vi "Cycle 0 Coast to Zero.vi"(0 "GEA2 Reference In":refnum<k24>, 5 "GEA Inputs":T1 {"Destination" format="%.0x"; "Source" format="%.0x"}, 7 "Standalone?":bool, 11 "Error In":errorcluster) -> (4 "GEA2 Reference Out":refnum<k24>, 6 "Pass/Fail?":bool, 8 "Report Text":string, 15 "Error Out":errorcluster)   [LabVIEW 2016, in "2015 VA Washer.lvlib"]
uses:
  Projects/2015 VA Washer.lvlib
  C:/Automation/DLLs/PC Dot Net/GeaCommunication.dll
  Common/LabVIEW GEA2 Toolkit/LabVIEW_GEA2_Toolkit.lvlibp/type defs/Source_Destination.ctl
  Valew Common/type defs/Drive Cycle Engine Request State.ctl
  Common/LabVIEW GEA2 Toolkit/LabVIEW_GEA2_Toolkit.lvlibp/type defs/ERD Read Data In.ctl
  Common/LabVIEW GEA2 Toolkit/LabVIEW_GEA2_Toolkit.lvlibp/type defs/Data Type.ctl
  Common/LabVIEW GEA2 Toolkit/LabVIEW_GEA2_Toolkit.lvlibp
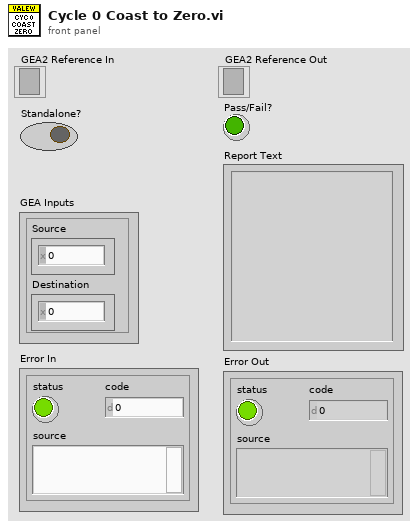
[diagram p1: front panel]
types:
  T1 = typedef "LabVIEW_GEA2_Toolkit.lvlibp/Source_Destination.ctl" = cluster{"Source":u8, "Destination":u8}
  T2 = typedef "2015 VA Washer.lvlib/Drive Cycle Engine Request State.ctl" = enum16{"Start", "Stop", "Pause", "Resume", "Select"}
  T3 = typedef "LabVIEW_GEA2_Toolkit.lvlibp/ERD Read Data In.ctl" = cluster{"ERD Number":u16, "Data Type":T4}
  T4 = typedef "LabVIEW_GEA2_Toolkit.lvlibp/Data Type.ctl" = enum16{"string", "boolean", "uint8_t", "uint16_t", "uint32_t", "uint64_t", "int8_t", "int16_t", "int32_t", "int64_t"}
  T5 = typedef "LabVIEW_GEA2_Toolkit.lvlibp/ERD Read Data Out.ctl" = cluster{"ERD Number":u16, "Data":string}
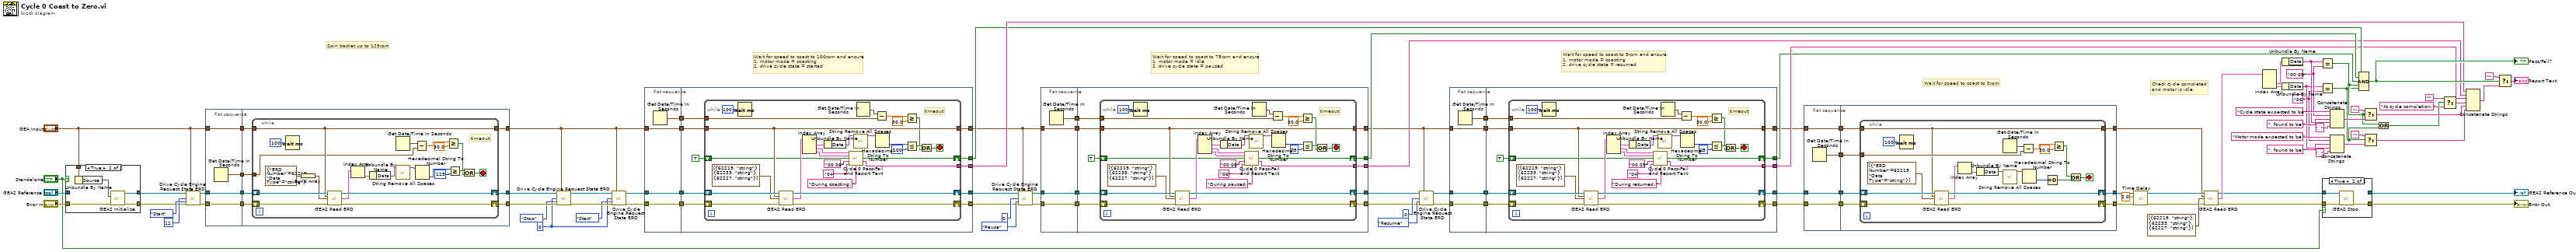
[diagram p0: block diagram]
diagram:
  w80 = "00 0B" ("y")
  w70 = "06" ("y")
  w93 = u8 0 ("Cycle ID")
  # "Check cycle completed\nand motor is idle"
  # "Wait for speed to coast to 0rpm"
  # "Wait for speed to coast to 5rpm and ensure\n1. motor mode = coasting\n2. drive cycle state = resumed"
  # "Wait for speed to coast to 75rpm and ensure\n1. motor mode = idle\n2. drive cycle state = paused"
  # "Wait for speed to coast to 100rpm and ensure\n1. motor mode = coasting\n2. drive cycle state = started"
  # "Spin basket up to 125rpm"
  n1 = case shown="True" "Standalone?" {
    tunnel: "GEA2 Reference In" -> [w104 _]
    tunnel: [w104 w109] -> w19
    tunnel: "Error In" -> [w103 w108]
    tunnel: [w103 w107] -> w17
    tunnel: "GEA Inputs" -> [_ w106]
    frame False {
    }
    frame True {
      n2 = Unbundle By Name(w106) -> ("Source"=w105:u8)
      n3 = call "GEA2 Initialize.vi"("Source Address"=w105, "error in"=w108) -> ("GEA2 Reference Out"=w109:refnum<k24>, "error out"=w107:errorcluster)  [unwired: 11 in, 1 out]
    }
  }
  n4 = call "Drive Cycle Engine Request State ERD.vi"("GEA2 Reference In"=w19, "GEA Inputs"="GEA Inputs", "Cycle ID"=u8 12, "Drive Cycle Engine Request State"=Drive_Cycle_Engine_Request_State."Start", "Error In"=w17) -> ("GEA2 Reference Out"=w99:refnum<k24>, "Error Out"=w100:errorcluster)  [unwired: 9 in]
  n5 = flat-sequence {
    tunnel: "GEA Inputs" -> [w111]
    tunnel: w99 -> [w112]
    tunnel: w100 -> [w113]
    tunnel: [w113] -> w91
    tunnel: [w112] -> w90
    tunnel: [w111] -> w89
    tunnel: [w110] -> w88
    tunnel: [w118] -> w98
    tunnel: [w117] -> w97
    tunnel: [w115] -> w49
    tunnel: w91 -> [w120]
    tunnel: w90 -> [w119]
    tunnel: w89 -> [w116]
    tunnel: w88 -> [w114]
    frame #0 {
      n6 = Get Date/Time In Seconds() -> (seconds since 1Jan1904=w110:timestamp)
    }
    frame #1 {
      n7 = while {
        shift-right: [w140] -> w117
        shift-left: w120 -> [w141]
        shift-right: [w138] -> w118
        shift-left: w119 -> [w139]
        tunnel: w116 -> [w131]
        tunnel: [w131] -> w115
        tunnel: w114 -> [w129]
        stop <- w126 stop-if-true
        # "timeout"
        n8 = Wait (ms)(milliseconds to wait=u32 100) -> ()  [unwired: 1 out]
        n9 = Build Array(T3 {"ERD Number"=62219, "Data Type"=enum."string"} ("ERD Read Data In")) -> (w137:T3[])
        n10 = call "GEA2 Read ERD.vi"("GEA2 Reference In"=w139, "GEA Inputs"=w131, "Read ERD List"=w137, "Error In"=w141) -> ("GEA2 Reference Out"=w138:refnum<k24>, "ERD Data Out"=w135:T5[], "Error Out"=w140:errorcluster)  [unwired: 8 in, 1 out]
        n11 = Index Array(array=w135) -> (element=w134:T5)  [unwired: 1 in]
        n12 = Unbundle By Name(w134) -> ("Data"=w121:string)
        n13 = Get Date/Time In Seconds() -> (seconds since 1Jan1904=w130:timestamp)
        n14 = call "String Remove All Spaces.vi"("Input String"=w121) -> ("Spaces Removed"=w122:string)  [unwired: 13 in, 1 out]
        n15 = Subtract(x=w130, y=w129) -> (x-y=w128:dbl)
        n16 = Hexadecimal String To Number(string=w122) -> (number=w133:u32)  [unwired: 2 in, 1 out]
        n17 = Greater Or Equal?(x=w128, y=30.0) -> (x >= y?=w124:bool)
        n18 = Greater Or Equal?(x=w133, y=u32 125) -> (x >= y?=w125:bool)
        n19 = Or(x=w125, y=w124) -> (x .or. y?=w126:bool)
      }
    }
  }
  n20 = call "Drive Cycle Engine Request State ERD.vi"("GEA2 Reference In"=w98, "GEA Inputs"=w49, "Cycle ID"=w93, "Drive Cycle Engine Request State"=Drive_Cycle_Engine_Request_State."Stop", "Error In"=w97) -> ("GEA2 Reference Out"=w95:refnum<k24>, "Error Out"=w94:errorcluster)  [unwired: 9 in]
  n21 = call "Drive Cycle Engine Request State ERD.vi"("GEA2 Reference In"=w95, "GEA Inputs"=w49, "Cycle ID"=w93, "Drive Cycle Engine Request State"=Drive_Cycle_Engine_Request_State."Start", "Error In"=w94) -> ("GEA2 Reference Out"=w50:refnum<k24>, "Error Out"=w51:errorcluster)  [unwired: 9 in]
  n22 = flat-sequence {
    tunnel: w51 -> [w143]
    tunnel: w49 -> [w144]
    tunnel: w50 -> [w145]
    tunnel: [w145] -> w55
    tunnel: [w144] -> w54
    tunnel: [w143] -> w53
    tunnel: [w142] -> w52
    tunnel: w55 -> [w155]
    tunnel: w54 -> [w154]
    tunnel: w53 -> [w153]
    tunnel: w52 -> [w152]
    tunnel: [w150] -> w47
    tunnel: [w149] -> w48
    tunnel: [w148] -> w38
    tunnel: [w147] -> w45
    tunnel: [w146] -> w46
    frame #0 {
      n23 = Get Date/Time In Seconds() -> (seconds since 1Jan1904=w142:timestamp)
    }
    frame #1 {
      n24 = while {
        shift-right: [w182] -> w150
        shift-left: w153 -> [w183]
        shift-right: [w180] -> w149
        shift-left: w155 -> [w181]
        tunnel: w154 -> [w177]
        tunnel: [w177] -> w148
        tunnel: w152 -> [w174]
        shift-right: [w160] -> w147
        shift-left: TRUE -> [w161]
        tunnel: [w159] -> w146
        stop <- w171 stop-if-true
        # "timeout"
        n25 = Wait (ms)(milliseconds to wait=u32 100) -> ()  [unwired: 1 out]
        n26 = call "GEA2 Read ERD.vi"("GEA2 Reference In"=w181, "GEA Inputs"=w177, "Read ERD List"=T3[] [{"ERD Number"=62219, "Data Type"=enum."string"}, {"ERD Number"=62233, "Data Type"=enum."string"}, {"ERD Number"=62227, "Data Type"=enum."string"}], "Error In"=w183) -> ("GEA2 Reference Out"=w180:refnum<k24>, "ERD Data Out"=w179:T5[], "Error Out"=w182:errorcluster)  [unwired: 8 in, 1 out]
        n27 = Index Array(array=w179) -> (element #1=w178:T5, element #2=w163:T5, element #3=w162:T5)  [unwired: 3 in]
        n28 = Unbundle By Name(w178) -> ("Data"=w166:string)
        n29 = call "Cycle 0 Pass-Fail and Report Text.vi"("Drive Cycle State"=w163, "Motor Mode"=w162, "Previous Pass/Fail"=w161, "Cycle State Expected"="00 06", "Motor Mode Expected"="04", "Header"="During coasting: ") -> ("Pass/Fail?"=w160:bool, "Report Text"=w159:string)  [unwired: 8 in]
        n30 = call "String Remove All Spaces.vi"("Input String"=w166) -> ("Spaces Removed"=w167:string)  [unwired: 13 in, 1 out]
        n31 = Get Date/Time In Seconds() -> (seconds since 1Jan1904=w173:timestamp)
        n32 = Subtract(x=w173, y=w174) -> (x-y=w175:dbl)
        n33 = Hexadecimal String To Number(string=w167) -> (number=w165:u32)  [unwired: 2 in, 1 out]
        n34 = Greater Or Equal?(x=w175, y=30.0) -> (x >= y?=w170:bool)
        n35 = Less Or Equal?(x=w165, y=u32 100) -> (x <= y?=w172:bool)
        n36 = Or(x=w172, y=w170) -> (x .or. y?=w171:bool)
      }
    }
  }
  n37 = call "Drive Cycle Engine Request State ERD.vi"("GEA2 Reference In"=w48, "GEA Inputs"=w38, "Cycle ID"=u8 0, "Drive Cycle Engine Request State"=Drive_Cycle_Engine_Request_State."Pause", "Error In"=w47) -> ("GEA2 Reference Out"=w39:refnum<k24>, "Error Out"=w40:errorcluster)  [unwired: 9 in]
  n38 = flat-sequence {
    tunnel: w40 -> [w185]
    tunnel: w38 -> [w186]
    tunnel: w39 -> [w187]
    tunnel: [w187] -> w44
    tunnel: [w186] -> w43
    tunnel: [w185] -> w42
    tunnel: [w184] -> w41
    tunnel: w44 -> [w197]
    tunnel: w43 -> [w196]
    tunnel: w42 -> [w195]
    tunnel: w41 -> [w194]
    tunnel: [w192] -> w35
    tunnel: [w191] -> w36
    tunnel: [w190] -> w28
    tunnel: [w189] -> w37
    tunnel: [w188] -> w21
    frame #0 {
      n39 = Get Date/Time In Seconds() -> (seconds since 1Jan1904=w184:timestamp)
    }
    frame #1 {
      n40 = while {
        shift-right: [w224] -> w192
        shift-left: w195 -> [w225]
        shift-right: [w222] -> w191
        shift-left: w197 -> [w223]
        tunnel: w196 -> [w219]
        tunnel: [w219] -> w190
        tunnel: w194 -> [w216]
        shift-right: [w202] -> w189
        shift-left: TRUE -> [w203]
        tunnel: [w201] -> w188
        stop <- w213 stop-if-true
        # "timeout"
        n41 = Wait (ms)(milliseconds to wait=u32 100) -> ()  [unwired: 1 out]
        n42 = call "GEA2 Read ERD.vi"("GEA2 Reference In"=w223, "GEA Inputs"=w219, "Read ERD List"=T3[] [{"ERD Number"=62219, "Data Type"=enum."string"}, {"ERD Number"=62233, "Data Type"=enum."string"}, {"ERD Number"=62227, "Data Type"=enum."string"}], "Error In"=w225) -> ("GEA2 Reference Out"=w222:refnum<k24>, "ERD Data Out"=w221:T5[], "Error Out"=w224:errorcluster)  [unwired: 8 in, 1 out]
        n43 = Index Array(array=w221) -> (element #1=w220:T5, element #2=w205:T5, element #3=w204:T5)  [unwired: 3 in]
        n44 = Unbundle By Name(w220) -> ("Data"=w208:string)
        n45 = call "Cycle 0 Pass-Fail and Report Text.vi"("Drive Cycle State"=w205, "Motor Mode"=w204, "Previous Pass/Fail"=w203, "Cycle State Expected"="00 08", "Motor Mode Expected"="06", "Header"="During paused: ") -> ("Pass/Fail?"=w202:bool, "Report Text"=w201:string)  [unwired: 8 in]
        n46 = call "String Remove All Spaces.vi"("Input String"=w208) -> ("Spaces Removed"=w209:string)  [unwired: 13 in, 1 out]
        n47 = Get Date/Time In Seconds() -> (seconds since 1Jan1904=w215:timestamp)
        n48 = Subtract(x=w215, y=w216) -> (x-y=w217:dbl)
        n49 = Hexadecimal String To Number(string=w209) -> (number=w207:u32)  [unwired: 2 in, 1 out]
        n50 = Greater Or Equal?(x=w217, y=30.0) -> (x >= y?=w212:bool)
        n51 = Less Or Equal?(x=w207, y=u32 75) -> (x <= y?=w214:bool)
        n52 = Or(x=w214, y=w212) -> (x .or. y?=w213:bool)
      }
    }
  }
  n53 = call "Drive Cycle Engine Request State ERD.vi"("GEA2 Reference In"=w36, "GEA Inputs"=w28, "Cycle ID"=u8 0, "Drive Cycle Engine Request State"=Drive_Cycle_Engine_Request_State."Resume", "Error In"=w35) -> ("GEA2 Reference Out"=w30:refnum<k24>, "Error Out"=w29:errorcluster)  [unwired: 9 in]
  n54 = flat-sequence {
    tunnel: w29 -> [w227]
    tunnel: w28 -> [w228]
    tunnel: w30 -> [w229]
    tunnel: [w229] -> w34
    tunnel: [w228] -> w33
    tunnel: [w227] -> w32
    tunnel: [w226] -> w31
    tunnel: w34 -> [w239]
    tunnel: w33 -> [w238]
    tunnel: w32 -> [w237]
    tunnel: w31 -> [w236]
    tunnel: [w234] -> w24
    tunnel: [w233] -> w25
    tunnel: [w232] -> w23
    tunnel: [w231] -> w26
    tunnel: [w230] -> w27
    frame #0 {
      n55 = Get Date/Time In Seconds() -> (seconds since 1Jan1904=w226:timestamp)
    }
    frame #1 {
      n56 = while {
        shift-right: [w266] -> w234
        shift-left: w237 -> [w267]
        shift-right: [w264] -> w233
        shift-left: w239 -> [w265]
        tunnel: w238 -> [w261]
        tunnel: [w261] -> w232
        tunnel: w236 -> [w258]
        shift-right: [w244] -> w231
        shift-left: TRUE -> [w245]
        tunnel: [w243] -> w230
        stop <- w255 stop-if-true
        # "timeout"
        n57 = Wait (ms)(milliseconds to wait=u32 100) -> ()  [unwired: 1 out]
        n58 = call "GEA2 Read ERD.vi"("GEA2 Reference In"=w265, "GEA Inputs"=w261, "Read ERD List"=T3[] [{"ERD Number"=62219, "Data Type"=enum."string"}, {"ERD Number"=62233, "Data Type"=enum."string"}, {"ERD Number"=62227, "Data Type"=enum."string"}], "Error In"=w267) -> ("GEA2 Reference Out"=w264:refnum<k24>, "ERD Data Out"=w263:T5[], "Error Out"=w266:errorcluster)  [unwired: 8 in, 1 out]
        n59 = Index Array(array=w263) -> (element #1=w262:T5, element #2=w247:T5, element #3=w246:T5)  [unwired: 3 in]
        n60 = Unbundle By Name(w262) -> ("Data"=w250:string)
        n61 = call "Cycle 0 Pass-Fail and Report Text.vi"("Drive Cycle State"=w247, "Motor Mode"=w246, "Previous Pass/Fail"=w245, "Cycle State Expected"="00 09", "Motor Mode Expected"="04", "Header"="During resumed: ") -> ("Pass/Fail?"=w244:bool, "Report Text"=w243:string)  [unwired: 8 in]
        n62 = call "String Remove All Spaces.vi"("Input String"=w250) -> ("Spaces Removed"=w251:string)  [unwired: 13 in, 1 out]
        n63 = Get Date/Time In Seconds() -> (seconds since 1Jan1904=w257:timestamp)
        n64 = Subtract(x=w257, y=w258) -> (x-y=w259:dbl)
        n65 = Hexadecimal String To Number(string=w251) -> (number=w249:u32)  [unwired: 2 in, 1 out]
        n66 = Greater Or Equal?(x=w259, y=30.0) -> (x >= y?=w254:bool)
        n67 = Less Or Equal?(x=w249, y=u32 15) -> (x <= y?=w256:bool)
        n68 = Or(x=w256, y=w254) -> (x .or. y?=w255:bool)
      }
    }
  }
  n69 = flat-sequence {
    tunnel: [w271] -> w65
    tunnel: w25 -> [w270]
    tunnel: [w270] -> w64
    tunnel: w24 -> [w269]
    tunnel: [w269] -> w63
    tunnel: w23 -> [w268]
    tunnel: [w268] -> w22
    tunnel: w65 -> [w278]
    tunnel: [w277] -> w2
    tunnel: [w276] -> w62
    tunnel: w64 -> [w275]
    tunnel: w63 -> [w274]
    tunnel: w22 -> [w273]
    tunnel: [w272] -> w10
    frame #0 {
      n70 = Get Date/Time In Seconds() -> (seconds since 1Jan1904=w271:timestamp)
    }
    frame #1 {
      n71 = while {
        shift-right: [w296] -> w277
        shift-left: w274 -> [w297]
        shift-right: [w294] -> w276
        shift-left: w275 -> [w295]
        tunnel: w278 -> [w289]
        tunnel: w273 -> [w279]
        tunnel: [w279] -> w272
        stop <- w287 stop-if-true
        n72 = Wait (ms)(milliseconds to wait=u32 100) -> ()  [unwired: 1 out]
        n73 = call "GEA2 Read ERD.vi"("GEA2 Reference In"=w295, "GEA Inputs"=w279, "Read ERD List"=T3[] [{"ERD Number"=62219, "Data Type"=enum."string"}], "Error In"=w297) -> ("GEA2 Reference Out"=w294:refnum<k24>, "ERD Data Out"=w293:T5[], "Error Out"=w296:errorcluster)  [unwired: 8 in, 1 out]
        n74 = Index Array(array=w293) -> (element=w292:T5)  [unwired: 1 in]
        n75 = Unbundle By Name(w292) -> ("Data"=w283:string)
        n76 = Get Date/Time In Seconds() -> (seconds since 1Jan1904=w288:timestamp)
        n77 = call "String Remove All Spaces.vi"("Input String"=w283) -> ("Spaces Removed"=w284:string)  [unwired: 13 in, 1 out]
        n78 = Subtract(x=w288, y=w289) -> (x-y=w290:dbl)
        n79 = Hexadecimal String To Number(string=w284) -> (number=w282:u32)  [unwired: 2 in, 1 out]
        n80 = Equal To 0?(x=w282) -> (x = 0?=w281:bool)
        n81 = Greater Or Equal?(x=w290, y=30.0) -> (x >= y?=w280:bool)
        n82 = Or(x=w280, y=w281) -> (x .or. y?=w287:bool)
      }
    }
  }
  n83 = call "Time Delay"("error in (no error)"=w2, "Delay Time (s)"=2.0) -> ("error out"=w1:errorcluster)  [unwired: 9 in]
  n84 = call "GEA2 Read ERD.vi"("GEA2 Reference In"=w62, "GEA Inputs"=w10, "Read ERD List"=T3[] [{"ERD Number"=62219, "Data Type"=enum."string"}, {"ERD Number"=62233, "Data Type"=enum."string"}, {"ERD Number"=62227, "Data Type"=enum."string"}], "Error In"=w1) -> ("GEA2 Reference Out"=w12:refnum<k24>, "ERD Data Out"=w84:T5[], "Error Out"=w14:errorcluster)  [unwired: 8 in, 1 out]
  n85 = Index Array(array=w84) -> (element #2=w87:T5, element #3=w86:T5)  [unwired: 3 in, 1 out]
  n86 = Unbundle By Name(w87) -> ("Data"=w78:string)
  n87 = Unbundle By Name(w86) -> ("Data"=w68:string)
  n88 = Equal?(x=w78, y=w80) -> (x = y?=w8:bool)
  n89 = Equal?(x=w68, y=w70) -> (x = y?=w7:bool)
  n90 = case shown="True" "Standalone?" {
    tunnel: [w298 w302] -> w15
    tunnel: w14 -> [w298 w301]
    tunnel: w12 -> [w299 w300]
    tunnel: [w299 _] -> w11
    frame False {
    }
    frame True {
      n91 = call "GEA2 Stop.vi"("GEA2 Reference In"=w300, "Error In"=w301) -> ("Error Out"=w302:errorcluster)  [unwired: 13 in]
    }
  }
  "GEA2 Reference Out" <- w11
  "Error Out" <- w15
  n92 = Concatenate Strings("Cycle state expected to be " ("string"), w80, ", found to be " ("string"), w78, ". " ("string")) -> (w76:string)
  n93 = Concatenate Strings("Motor mode expected to be " ("string"), w70, ", found to be " ("string"), w68, ". " ("string")) -> (w73:string)
  n94 = Compound Arithmetic op=AND(w45, w37, w26, w8, w7) -> (w83:bool)
  "Pass/Fail?" <- w83
  n95 = Select(t="", s=w8, f=w76) -> (s? t:f=w61:string)
  n96 = Select(t="", s=w7, f=w73) -> (s? t:f=w60:string)
  n97 = Or(x=w8, y=w7) -> (x .or. y?=w6:bool)
  n98 = Select(t="", s=w6, f="At cycle completion: " ("string")) -> (s? t:f=w9:string)
  n99 = Concatenate Strings(w46, w21, w27, w9, w61, w60) -> (w72:string)
  n100 = Select(t="", s=w83, f=w72) -> (s? t:f=→"Report Text":string)
